vi "Stop Animation.vi"(8 "Error In":errorcluster, 11 "Animation Config":T1) -> (0 "Error Out":errorcluster)   [LabVIEW 2011, in "LVH-Toolbox.lvlib" / "GUI Tools.lvlib"]
uses:
  GUI Tools.lvlib
  Private/Animations/Type Defs/Animation Config.ctl
  <vilib>/picture/picture.llb/imagedata.ctl
  Private/Animations/FGVs/Type Defs/Animation FGV State.ctl
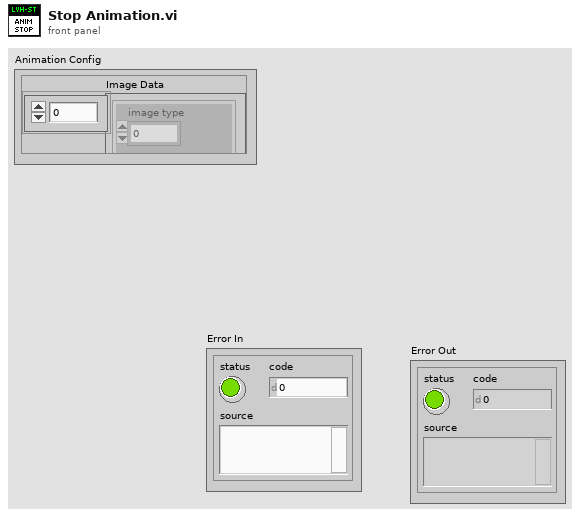
[diagram p1: front panel]
types:
  T1 = typedef "LVH-Toolbox.lvlib/GUI Tools.lvlib/Animation Config.ctl" = cluster{"Image Data":T2[], "Animation Picture Indicator":refnum<vi>, "FPS":u32, "Position":cluster{"X":i16, "Y":i16}}
  T2 = typedef "imagedata.ctl" = cluster{"image type":i32, "image depth":i32, "image":u8[], "mask":u8[], "colors":u32[], "Rectangle":cluster{"left":i16, "top":i16, "right":i16, "bottom":i16}}
  T3 = typedef "LVH-Toolbox.lvlib/GUI Tools.lvlib/Animation FGV State.ctl" = enum16{"Init", "Set", "Get"}
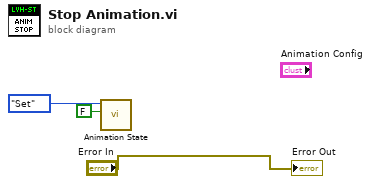
[diagram p0: block diagram]
diagram:
  n1 = call "Animation State.vi"("Running?"=FALSE, "Function"=Animation_FGV_State."Set") -> ()  [unwired: 9 in, 1 out]
  "Error Out" <- "Error In"
